vi "End.vi"(8 "error in (no error)":errorcluster, 11 "Simulated_CCD_Camera in":refnum<class "Sim_CCD.lvclass">) -> (0 "error out":errorcluster, 3 "Simulated_CCD_Camera out":refnum<class "Sim_CCD.lvclass">)   [LabVIEW 2018, in "Sim_CCD.lvclass"]
doc: "Correctly ends communication with the camera."
uses:
  Sim_CCD.lvclass
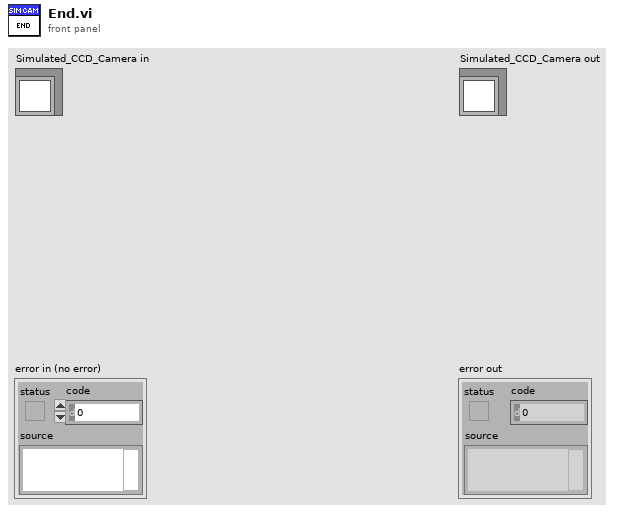
[diagram p1: front panel]
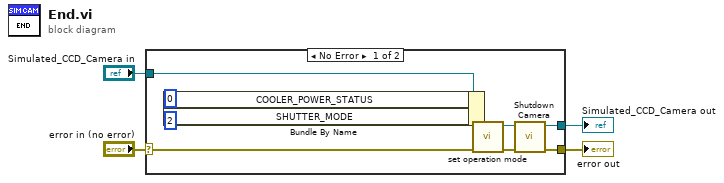
[diagram p0: block diagram]
diagram:
  n1 = case shown="No Error" "error in (no error)" {
    selector: "error in (no error)" -> [w8 w15]
    tunnel: [w12 w15] -> w3
    tunnel: [w11 w14] -> w1
    tunnel: "Simulated_CCD_Camera in" -> [w10 w14]
    frame No Error {
      n2 = Bundle By Name(cluster=w10, "COOLER_POWER_STATUS"=u16 0, "SHUTTER_MODE"=u16 2 ("New CCD Config.SHUTTER_MODE")) -> (w5:refnum<class "Sim_CCD.lvclass">)
      n3 = call-dynamic "set operation mode.vi"("error in (no error)"=w8, "CCDCamera in"=w5) -> ("error out"=w6:errorcluster, "CCDCamera out"=w7:refnum<class "Sim_CCD.lvclass">)  [unwired: 8 in]
      n4 = call-dynamic "Shutdown Camera.vi"("error in (no error)"=w6, "CCDCamera in"=w7) -> ("error out"=w12:errorcluster, "CCDCamera out"=w11:refnum<class "Sim_CCD.lvclass">)  [unwired: 8 in]
    }
    frame Error {
    }
  }
  "error out" <- w3
  "Simulated_CCD_Camera out" <- w1
